vi "Pre Launch Init.vi"(11 "Humidifier in":refnum<class "Humidifier.lvclass">) -> (0 "error out":errorcluster, 3 "Humidifier out":refnum<class "Humidifier.lvclass">)   [LabVIEW 2014, in "Humidifier Lib.lvlib" / "Humidifier.lvclass"]
doc: "(<B>Filename</B>: Actor Framework.lvlib:Actor.lvclass:Pre Launch Init.vi)\n\nDefines behavior that occurs after the Launch Nested Actor method is invoked but before the actor's Actor Core method begins running.\n\nBy default, this method does nothing. A descendant class may override it to define behavior."
uses:
  Humidifier.lvclass
  Humidifier.lvclass/Humidifier.ctl
  reusable/Command/Command.lvclass
  reusable/Session APIs/File Access/Config Data/Config Data.lvclass
  reusable/Session APIs/File Access/Config Data/Config Data.lvclass/Config Data.ctl
  reusable/Session APIs/File Access/Config Data/Accessors/Read Ref.vi
  <vilib>/Utility/config.llb/Read Key (String).vi
  <vilib>/Utility/config.llb/Read Key (Boolean).vi
  <vilib>/Utility/config.llb/Read Key (Double).vi
  <vilib>/Utility/config.llb/NI_LVConfig.lvlib
  <userlib>/_Session Fwk/Session - Root.lvclass
  reusable/Session APIs/Session Log/System Log.lvclass
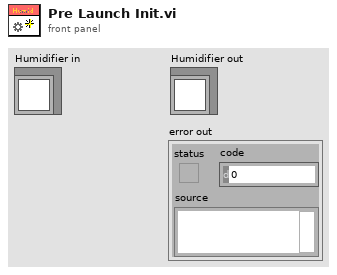
[diagram p1: front panel]
types:
  T1 = typedef "Session - Root.lvclass/Session Handle.ctl" = refnum<data-value>
  T2 = typedef "NI_LVConfig.lvlib/Config Data RefNum.ctl" = refnum<k1>
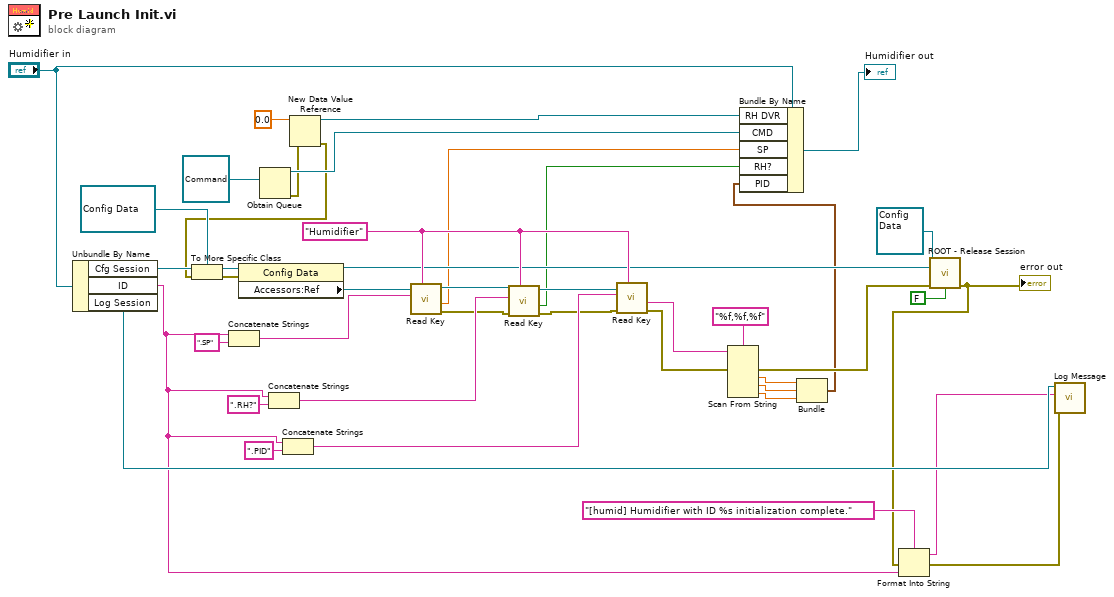
[diagram p0: block diagram]
diagram:
  w26 = "Humidifier" ("section")
  n1 = Unbundle By Name("Humidifier in") -> ("Cfg Session"=w37:T1, "ID"=w4:string, "Log Session"=w6:T1)
  n2 = Concatenate Strings(w4, ".SP" ("string")) -> (w31:string)
  n3 = Obtain Queue(element data type=refnum<class "Command.lvclass"> refnum ("CMD")) -> (queue out=w39:refnum<queue>, error out=w8:errorcluster)  [unwired: 4 in, 1 out]
  n4 = Concatenate Strings(w4, ".RH?" ("string")) -> (w29:string)
  n5 = Concatenate Strings(w4, ".PID" ("string")) -> (w24:string)
  n6 = New Data Value Reference(data value=sgl 0.0 ("Current RH"), error in=w8) -> (data value reference=w42:refnum<data-value>, error out=w7:errorcluster)
  n7 = To More Specific Class(target class=refnum<data-value> refnum ("Session Handle"), reference=w37, error in=w7) -> (specific class reference=w35:refnum<data-value>, error out=w33:errorcluster)
  n8 = property class="Config Data"(reference=w35, error in=w33) -> (reference out=w18:refnum<data-value>, "Accessors:Ref"=w34:T2)  [unwired: 1 out]
  n9 = call-poly <vilib>:"Read Key.vi"("section"=w26, "key"=w31, "refnum"=w34) -> ("error out"=w19:errorcluster, "value"=w13:dbl, "refnum out"=w28:T2)  [unwired: 5 in, 1 out]
  n10 = call-poly <vilib>:"Read Key.vi"("section"=w26, "error in (no error)"=w19, "key"=w29, "refnum"=w28) -> ("error out"=w20:errorcluster, "value"=w12:bool, "refnum out"=w27:T2)  [unwired: 4 in, 1 out]
  n11 = call-poly <vilib>:"Read Key.vi"("section"=w26, "error in (no error)"=w20, "key"=w24, "refnum"=w27) -> ("error out"=w21:errorcluster, "value"=w23:string)  [unwired: 4 in, 2 out]
  n12 = Scan From String(format string="%f,%f,%f", input string=w23, error in=w21) -> (error out=w17:errorcluster, output 1=w16:dbl, output 2=w15:dbl, output 3=w14:dbl)  [unwired: 4 in, 2 out]
  n13 = Bundle(w16, w15, w14) -> (w11:cluster{dbl, dbl, dbl})  [unwired: 1 in]
  n14 = Bundle By Name(cluster="Humidifier in", "RH DVR"=w42, "CMD"=w39, "SP"=w13, "RH?"=w12, "PID"=w11) -> (→"Humidifier out":refnum<class "Humidifier.lvclass">)
  n15 = call <userlib>:"ROOT - Release Session.vi"("OBJ - Session in"=refnum<class "Config Data.lvclass"> refnum ("Config Data"), "Session Handle in"=w18, "error in (no error)"=w17, "force destroy? (F)"=FALSE) -> ("error out"=w1:errorcluster)  [unwired: 10 in, 1 out]
  "error out" <- w1
  n16 = Format Into String(format string="[humid] Humidifier with ID %s initialization complete." ("MSG In"), error in=w1, w4) -> (resulting string=w3:string, error out=w2:errorcluster)  [unwired: 1 in]
  n17 = call "Log Message.vi"("error in"=w2, "MSG In"=w3, "session in"=w6) -> ()  [unwired: 7 in, 2 out]
